vi "Main - Intilization.vi"(8 "Error In":errorcluster, 11 "Exe Name":string="VSys DAQ") -> (0 "Error Out":errorcluster)   [LabVIEW 2020]
uses:
  Control/State - FGV.ctl
  <vilib>/Utility/sysdir.llb/System Directory Type.ctl
  <vilib>/Utility/config.llb/Write Key (Boolean).vi
  <vilib>/Utility/config.llb/NI_LVConfig.lvlib
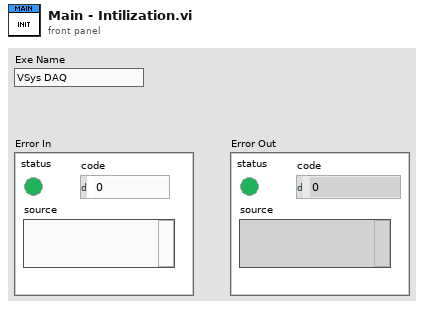
[diagram p1: front panel]
types:
  T1 = enum16{"Init Path", "Create Folder", "Create Folder Log", "Init System Path", "Create Config File", "Init Variables", "Read Page Configuration", "Close"}
  T2 = typedef "State - FGV.ctl" = enum16{"Write", "Read"}
  T3 = enum32{"invalid app kind", "Development System", "Run Time System", "Student Edition", "Embedded LabVIEW", "Evaluation", "Custom"}
  T4 = typedef "System Directory Type.ctl" = i32
  T5 = typedef "NI_LVConfig.lvlib/Config Data RefNum.ctl" = refnum<k1>
  T6 = typedef "License File Parameter.ctl" = cluster{"Expired Time":string, "Computer ID":string, "Product Name":string, "Period":i16, "Activated Time":string, "License Level":enum16{"Level 1", "Level 2", "Level 3", "Level 4", "Level 5"}, "License Type":enum16{"Free", "Trial", "Subscription", "Perpetual"}, "Log Time":string}
  T7 = enum16{"Level 1", "Level 2", "Level 3", "Level 4", "Level 5"}
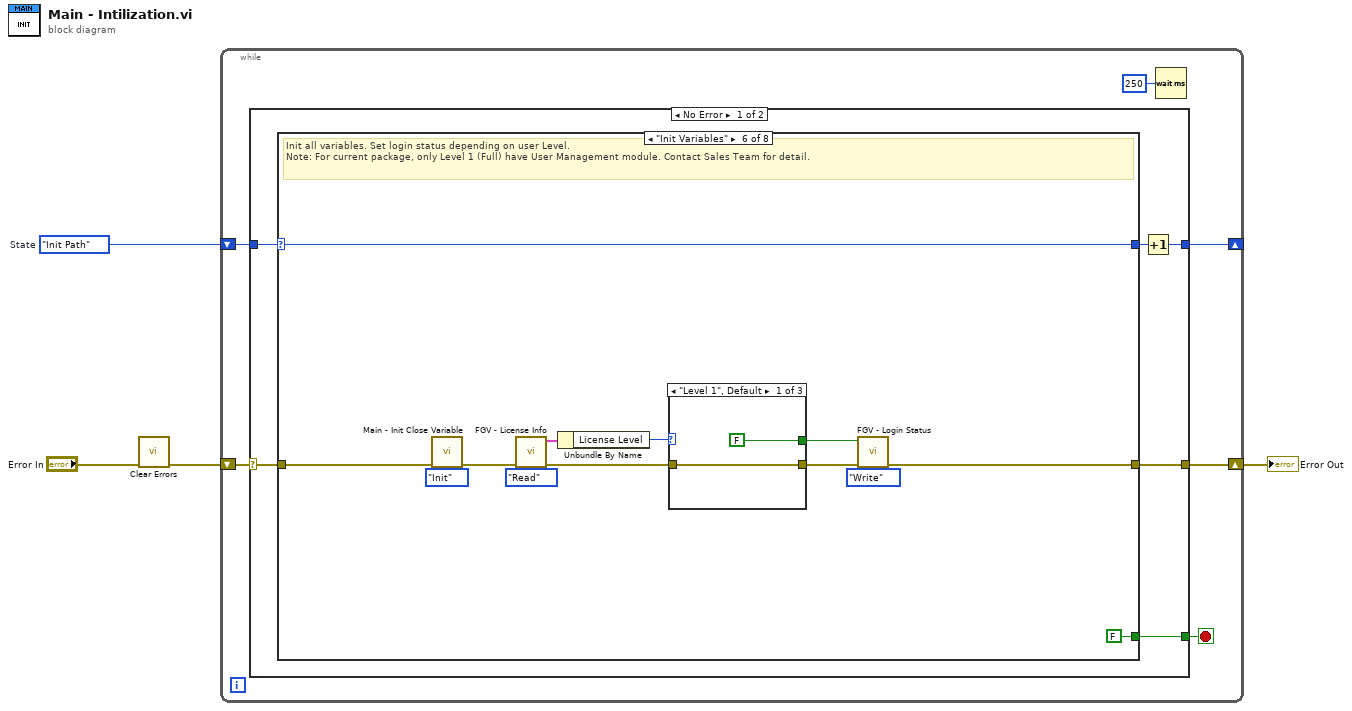
[diagram p0: block diagram]
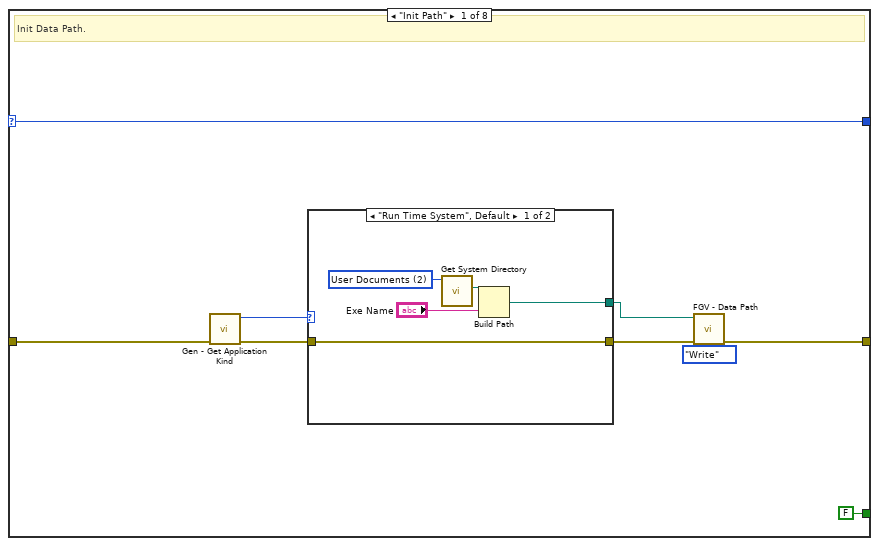
[diagram p2: hidden frame]
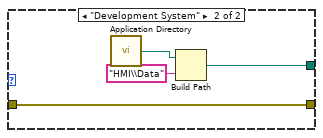
[diagram p3: hidden frame]
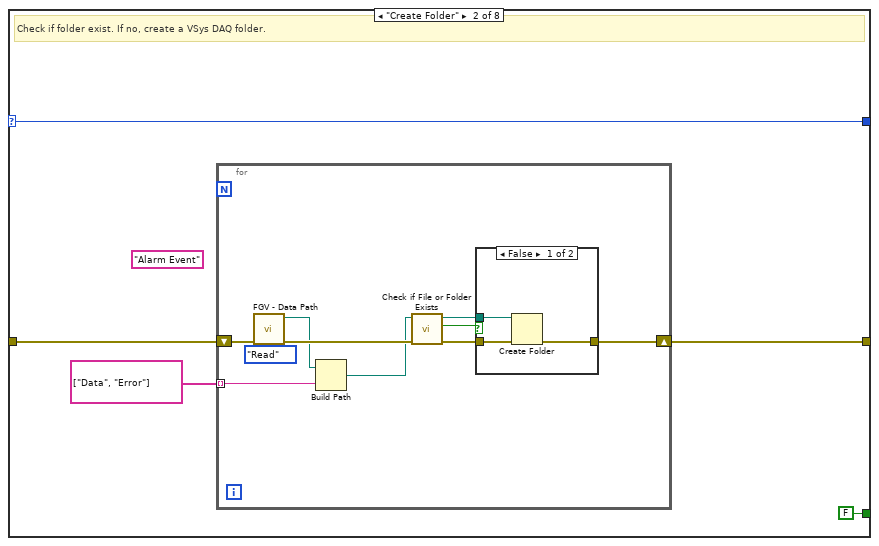
[diagram p4: hidden frame]
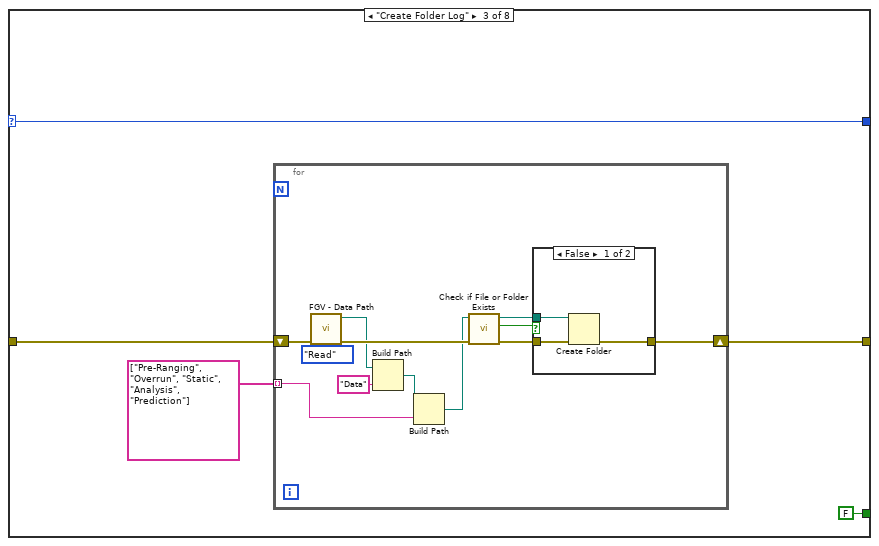
[diagram p6: hidden frame]
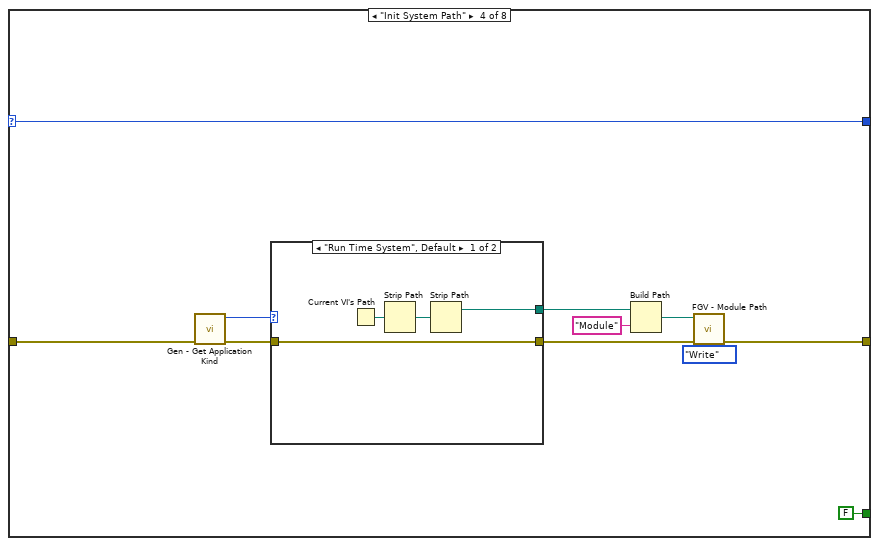
[diagram p8: hidden frame]
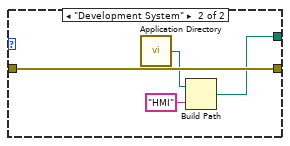
[diagram p9: hidden frame]
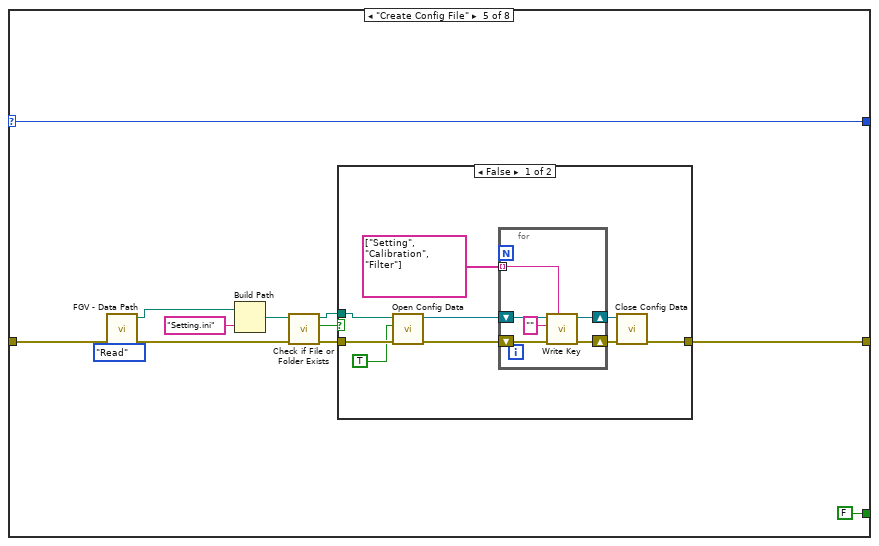
[diagram p10: hidden frame]
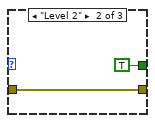
[diagram p12: hidden frame]
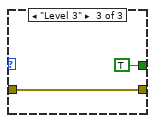
[diagram p13: hidden frame]
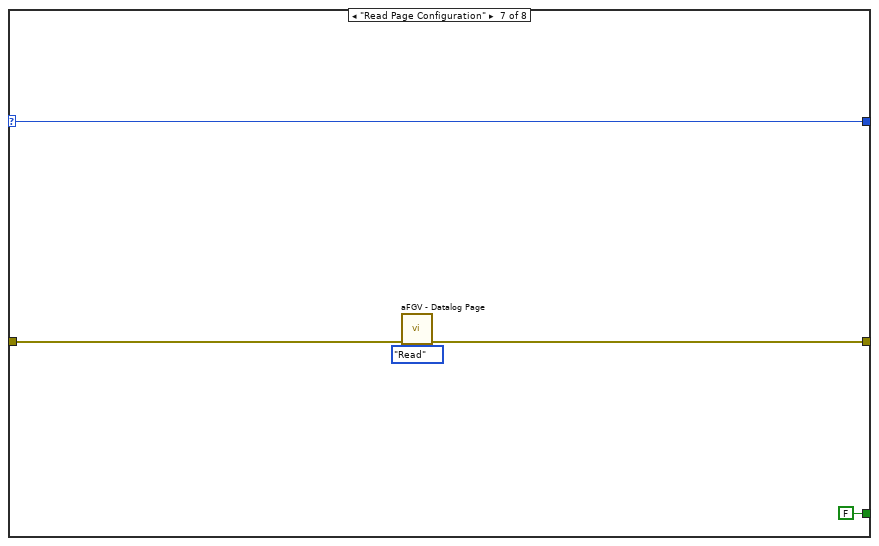
[diagram p14: hidden frame]
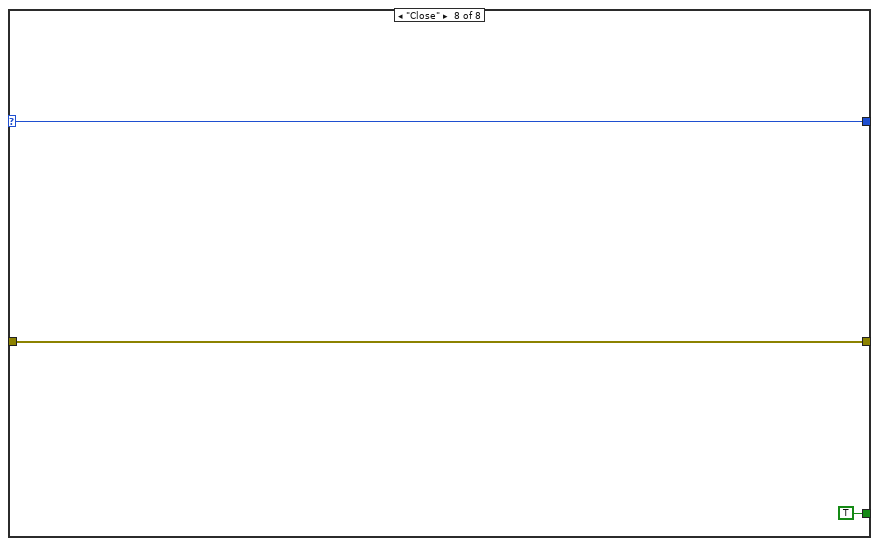
[diagram p15: hidden frame]
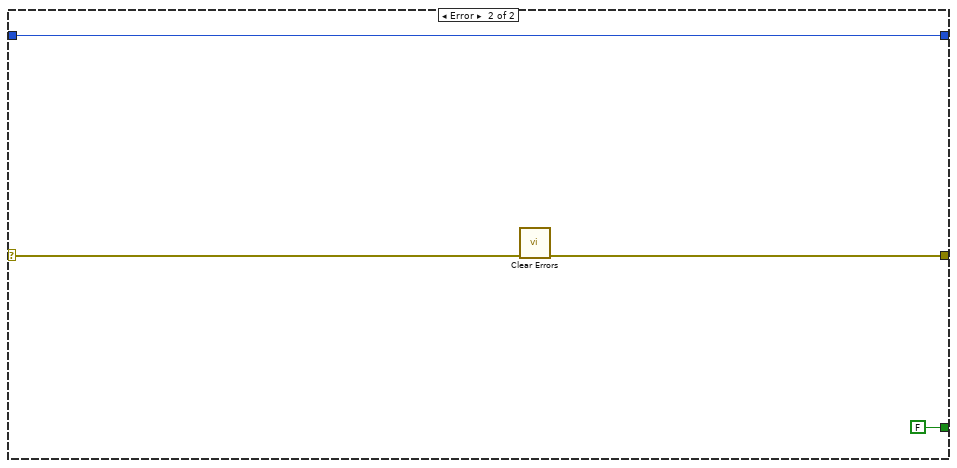
[diagram p16: hidden frame]
diagram:
  w1 = T1."Init Path"  # State
  n1 = call <vilib>:"Clear Errors.vi"("error in (no error)"="Error In") -> ("error out"=w2:errorcluster)  [unwired: 5 in, 1 out]
  n2 = while {
    shift-right: [w9] -> w3
    shift-left: w2 -> [w10]
    shift-right: [w6] -> _
    shift-left: w1 -> [w8]
    stop <- w7 stop-if-true
    n3 = case shown="No Error" w10 {
      selector: w10 -> [w15 w152]
      tunnel: [w16 w151] -> w9
      tunnel: w8 -> [w14 w149]
      tunnel: [w11 FALSE] -> w7
      tunnel: [w12 w149] -> w6
      frame No Error {
        n4 = case shown="\"Init Variables\"" w14 {
          selector: w14 -> [w21 w37 w54 w81 w101 w129 w143 w147]
          tunnel: [w24 w38 w57 w85 w103 w132 w144 w148] -> w16
          tunnel: w15 -> [w23 w39 w58 w84 w105 w134 w145 w148]
          tunnel: [w21 w37 w54 w81 w101 w129 w143 w147] -> w13
          tunnel: [FALSE FALSE FALSE FALSE FALSE FALSE FALSE TRUE] -> w11
          frame "Init Path" {
            # "Init Data Path."
            n5 = call "Gen - Get Application Kind.vi"("Error In"=w23) -> ("Error Out"=w22:errorcluster, "Application:Kind"=w18:T3)  [unwired: 9 in]
            n6 = case shown="\"Run Time System\", Default" w18 {
              tunnel: [w30 w34] -> w25
              tunnel: w22 -> [w30 w34]
              tunnel: [w26 w31] -> w17
              frame "Run Time System", Default {
                w29 = T4 2 items=["User Home"=0, "User Desktop"=1, "User Documents"=2, "User Application Data"=3, "User Preferences"=4, "User Temporary"=5, "Public Documents"=6, "Public Application Data"=7, "Public Preferences"=8, "Public Cache"=13, "System Core Libraries"=9, "System Installed Libraries"=10, "Application Files"=11, "Boot Volume Root"=12] ("system directory type")
                n7 = call <vilib>:"Get System Directory.vi"("system directory type"=w29) -> ("system directory"=w27:path)  [unwired: 10 in]
                n8 = Build Path(base path=w27, name or relative path="Exe Name") -> (appended path=w26:path)
              }
              frame "Development System" {
                n9 = call <vilib>:"Application Directory.vi"() -> ("Application Directory"=w33:path)
                n10 = Build Path(base path=w33, name or relative path="HMI\\Data") -> (appended path=w31:path)
              }
            }
            n11 = call "FGV - Data Path.vi"("FGV State"=State_-_FGV."Write", "Error In"=w25, "Path In"=w17) -> ("Error Out"=w24:errorcluster)  [unwired: 7 in, 1 out]
          }
          frame "Create Folder" {
            (unwired) "Alarm Event" ("name or relative path")
            # "Check if folder exist. If no, create a VSys DAQ folder."
            n12 = for {
              tunnel: string[] ["Data", "Error"] ("name or relative path") -> [w44] mode=indexing
              shift-right: [w46] -> w38
              shift-left: w39 -> [w49]
              n13 = call "FGV - Data Path.vi"("FGV State"=State_-_FGV."Read", "Error In"=w49) -> ("Error Out"=w48:errorcluster, "Path Out"=w43:path)  [unwired: 8 in]
              n14 = Build Path(base path=w43, name or relative path=w44) -> (appended path=w42:path)
              n15 = call <vilib>:"Check if File or Folder Exists.vi"("error in (no error)"=w48, "path"=w42) -> ("error out"=w47:errorcluster, "file or folder exists?"=w40:bool, "dup path"=w41:path)  [unwired: 7 in]
              n16 = case shown="False" w40 {
                tunnel: w47 -> [w52 w53]
                tunnel: [w51 w53] -> w46
                tunnel: w41 -> [w50 _]
                frame False {
                  n17 = Create Folder(path (use dialog)=w50, error in=w52) -> (error out=w51:errorcluster)  [unwired: 1 in, 2 out]
                }
                frame True {
                }
              }
            }
          }
          frame "Create Folder Log" {
            n18 = for {
              tunnel: string[] ["Pre-Ranging", "Overrun", "Static", "Analysis", "Prediction"] ("name or relative path") -> [w59] mode=indexing
              shift-right: [w67] -> w57
              shift-left: w58 -> [w70]
              n19 = call "FGV - Data Path.vi"("FGV State"=State_-_FGV."Read", "Error In"=w70) -> ("Error Out"=w69:errorcluster, "Path Out"=w65:path)  [unwired: 8 in]
              n20 = Build Path(base path=w65, name or relative path="Data") -> (appended path=w61:path)
              n21 = Build Path(base path=w61, name or relative path=w59) -> (appended path=w60:path)
              n22 = call <vilib>:"Check if File or Folder Exists.vi"("error in (no error)"=w69, "path"=w60) -> ("error out"=w68:errorcluster, "file or folder exists?"=w63:bool, "dup path"=w64:path)  [unwired: 7 in]
              n23 = case shown="False" w63 {
                tunnel: w68 -> [w73 w74]
                tunnel: [w72 w74] -> w67
                tunnel: w64 -> [w71 _]
                frame False {
                  n24 = Create Folder(path (use dialog)=w71, error in=w73) -> (error out=w72:errorcluster)  [unwired: 1 in, 2 out]
                }
                frame True {
                }
              }
            }
          }
          frame "Init System Path" {
            n25 = call "Gen - Get Application Kind.vi"("Error In"=w84) -> ("Error Out"=w83:errorcluster, "Application:Kind"=w76:T3)  [unwired: 9 in]
            n26 = case shown="\"Run Time System\", Default" w76 {
              tunnel: [w88 w90] -> w77
              tunnel: [w89 w93] -> w82
              tunnel: w83 -> [w89 w93]
              frame "Run Time System", Default {
                n27 = Current VI's Path() -> (path=w87:path)
                n28 = Strip Path(path=w87) -> (stripped path=w86:path)  [unwired: 1 out]
                n29 = Strip Path(path=w86) -> (stripped path=w88:path)  [unwired: 1 out]
              }
              frame "Development System" {
                n30 = call <vilib>:"Application Directory.vi"() -> ("Application Directory"=w91:path)
                n31 = Build Path(base path=w91, name or relative path="HMI") -> (appended path=w90:path)
              }
            }
            n32 = Build Path(base path=w77, name or relative path="Module") -> (appended path=w75:path)
            n33 = call "FGV - Module Path.vi"("FGV State"=State_-_FGV."Write", "Error In"=w82, "Path In"=w75) -> ("Error Out"=w85:errorcluster)  [unwired: 7 in, 1 out]
          }
          frame "Create Config File" {
            n34 = call "FGV - Data Path.vi"("FGV State"=State_-_FGV."Read", "Error In"=w105) -> ("Error Out"=w104:errorcluster, "Path Out"=w97:path)  [unwired: 8 in]
            n35 = Build Path(base path=w97, name or relative path="Setting.ini") -> (appended path=w96:path)
            n36 = call <vilib>:"Check if File or Folder Exists.vi"("error in (no error)"=w104, "path"=w96) -> ("error out"=w102:errorcluster, "file or folder exists?"=w95:bool, "dup path"=w94:path)  [unwired: 7 in]
            n37 = case shown="False" w95 {
              tunnel: [w111 w121] -> w103
              tunnel: w102 -> [w112 w121]
              tunnel: w94 -> [w109 _]
              frame False {
                n38 = call <vilib>:"Open Config Data.vi"("error in (no error)"=w112, "create file if necessary (T)"=TRUE, "configuration file path"=w109) -> ("error out"=w114:errorcluster, "refnum"=w108:T5)  [unwired: 6 in, 1 out]
                n39 = for {
                  shift-right: [w117] -> w107
                  shift-left: w108 -> [w118]
                  shift-right: [w119] -> w113
                  shift-left: w114 -> [w120]
                  tunnel: string[] ["Setting", "Calibration", "Filter"] ("name or relative path") -> [w116] mode=indexing
                  n40 = call-poly <vilib>:"Write Key.vi"("section"=w116, "error in (no error)"=w120, "key"="", "refnum"=w118) -> ("error out"=w119:errorcluster, "refnum out"=w117:T5)  [unwired: 5 in, 1 out]
                }
                n41 = call <vilib>:"Close Config Data.vi"("error in (no error)"=w113, "refnum"=w107) -> ("error out"=w111:errorcluster)  [unwired: 8 in, 1 out]
              }
              frame True {
              }
            }
          }
          frame "Init Variables" {
            # "Init all variables. Set login status depending on user Level. \nNote: For current package, only Level 1 (Full) have User Management module. Contact Sales Team for detail."
            n42 = call "Main - Init Close Variable.vi"("State"=enum16{"Init", "Close"}."Init", "Error In"=w134) -> ("Error Out"=w133:errorcluster)  [unwired: 9 in]
            n43 = call "FGV - License Info.vi"("FGV States"=enum16{"Read", "Write"}."Read", "Error In"=w133) -> ("Error Out"=w131:errorcluster, "License Info"=w124:T6)  [unwired: 8 in]
            n44 = Unbundle By Name(w124) -> ("License Level"=w123:T7)
            n45 = case shown="\"Level 1\", Default" w123 {
              tunnel: [w136 w138 w140] -> w130
              tunnel: w131 -> [w136 w138 w140]
              tunnel: [FALSE TRUE TRUE] -> w122
              frame "Level 1", Default {
              }
              frame "Level 2" {
              }
              frame "Level 3" {
              }
            }
            n46 = call "FGV - Login Status.vi"("Action"=enum16{"Read", "Write"}."Write", "Error In"=w130, "Login In"=w122) -> ("Error Out"=w132:errorcluster)  [unwired: 6 in, 2 out]
          }
          frame "Read Page Configuration" {
            n47 = call "aFGV - Datalog Page.vi"("Action"=enum16{"Read", "Write"}."Read", "Error In"=w145) -> ("Error Out"=w144:errorcluster)  [unwired: 8 in, 1 out]
          }
          frame "Close" {
          }
        }
        n48 = Increment(x=w13) -> (x+1=w12:T1)
      }
      frame Error {
        n49 = call <vilib>:"Clear Errors.vi"("error in (no error)"=w152) -> ("error out"=w151:errorcluster)  [unwired: 5 in, 1 out]
      }
    }
    n50 = Wait (ms)(milliseconds to wait=u32 250) -> ()  [unwired: 1 out]
  }
  "Error Out" <- w3
